vi "Check Expiration.vi"(8 "error in (no error)":errorcluster, 10 "registered claims":T2, 11 "token creation":timestamp) -> (0 "error out":errorcluster, 2 "datetime valid":bool, 3 "date/time claims":T1)   [LabVIEW 2017, in "JSONWebToken.lvclass"]
uses:
  JSONWebToken.lvclass
  JWT registered Claims -- cluster.ctl
  <vilib>/LabVIEW Open Source Project/Epoch Date & Time/epoch.UNIX/Epoch.UNIX.lvclass
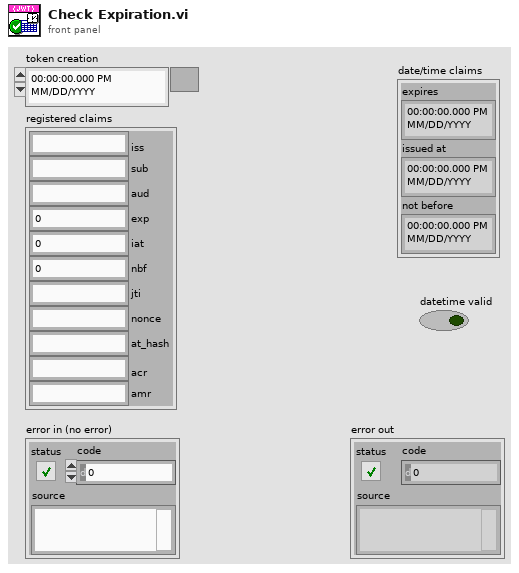
[diagram p1: front panel]
types:
  T1 = cluster{"expires":timestamp, "issued at":timestamp, "not before":timestamp}
  T2 = typedef "JSONWebToken.lvclass/JWT registered Claims -- cluster.ctl" = cluster{"iss":string, "sub":string, "aud":string, "exp":i32, "iat":i32, "nbf":i32, "jti":string, "nonce":string, "at_hash":string, "acr":string, "amr":string}
  T3 = cluster{"Timestamp":timestamp, "Timestamp":timestamp, "Timestamp":timestamp}
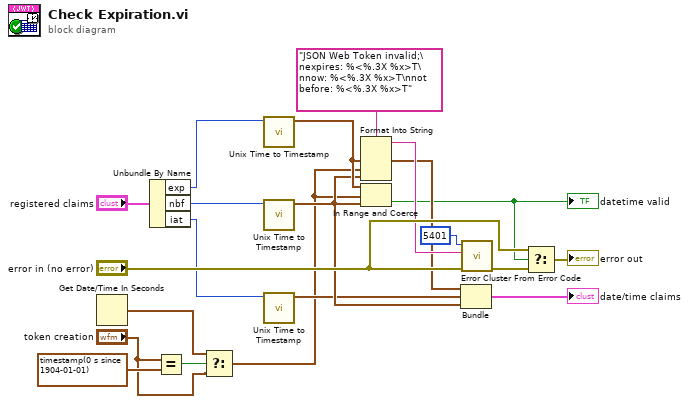
[diagram p0: block diagram]
diagram:
  n1 = Get Date/Time In Seconds() -> (seconds since 1Jan1904=w3:timestamp)
  n2 = Unbundle By Name("registered claims") -> ("exp"=w12:i32, "nbf"=w13:i32, "iat"=w11:i32)
  n3 = Equal?(x="token creation", y=timestamp(0 s since 1904-01-01) ("token creation")) -> (x = y?=w4:bool)
  n4 = Select(t=w3, s=w4, f="token creation") -> (s? t:f=w1:timestamp)
  n5 = call <vilib>:"Unix Time to Timestamp.vi"("Unix Time (s)"=w12) -> ("Timestamp"=w10:timestamp)  [unwired: 9 in, 1 out]
  n6 = call <vilib>:"Unix Time to Timestamp.vi"("Unix Time (s)"=w13) -> ("Timestamp"=w9:timestamp)  [unwired: 9 in, 1 out]
  n7 = call <vilib>:"Unix Time to Timestamp.vi"("Unix Time (s)"=w11) -> ("Timestamp"=w7:timestamp)  [unwired: 9 in, 1 out]
  n8 = Format Into String(format string="JSON Web Token invalid;\nexpires: %<%.3X %x>T\nnow: %<%.3X %x>T\nnot before: %<%.3X %x>T", w10, w1, w9) -> (resulting string=w15:string)  [unwired: 2 in, 1 out]
  n9 = In Range and Coerce(upper limit=w10, x=w1, lower limit=w9) -> (In Range?=w6:bool)  [unwired: 1 out]
  "datetime valid" <- w6
  n10 = Bundle("Timestamp"=w10, "Timestamp"=w7, "Timestamp"=w9) -> (→"date/time claims":T3)  [unwired: 1 in]
  n11 = call <vilib>:"Error Cluster From Error Code.vi"("error in (no error)"="error in (no error)", "error message (\"\")"=w15, "error code (0)"=5401) -> ("error out"=w18:errorcluster)  [unwired: 6 in]
  n12 = Select(t="error in (no error)", s=w6, f=w18) -> (s? t:f=→"error out":errorcluster)
